vi "Transport To Actor Type.vi"(10 "Spawn":refnum<class "Spawn.lvclass">) -> (2 "Actor Type":T1)   [LabVIEW 2025, in "jettl.lvlib" / "Actor.lvlib"]
uses:
  Actor.lvlib
  Actor Type.ctl
  Transport/Queue/Queue.lvlib
  Transport/Event/Event.lvlib
  Transport/Notifier/Notifier.lvlib
  Spawn/Spawn/Spawn.lvclass
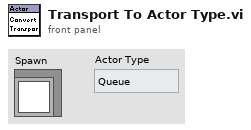
[diagram p1: front panel]
types:
  T1 = typedef "jettl.lvlib/Actor.lvlib/Actor Type.ctl" = enum16{"Queue", "Event", "Notifier"}
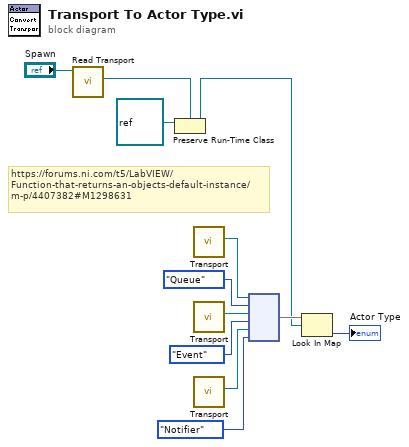
[diagram p0: block diagram]
diagram:
  # "https://forums.ni.com/t5/LabVIEW/Function-that-returns-an-objects-default-instance/m-p/4407382#M1298631"
  n1 = call-dynamic "Read Transport.vi"("Spawn in"="Spawn") -> ("Transport"=w2:refnum<class "Transport.lvclass">)  [unwired: 10 in]
  n2 = Preserve Run-Time Class(object in=refnum<class> refnum ("LabVIEW Object"), 2:w2) -> (object out=w4:refnum<class "Transport.lvclass">)  [unwired: 1 in, 1 out]
  n3 = call "Transport.vi"() -> ("Transport"=w12:refnum<class "Transport.lvclass">)  [unwired: 11 in]
  n4 = call "Transport.vi"() -> ("Transport"=w10:refnum<class "Transport.lvclass">)  [unwired: 11 in]
  n5 = call "Transport.vi"() -> ("Transport"=w9:refnum<class "Transport.lvclass">)  [unwired: 11 in]
  n6 = node(w12, Actor_Type."Queue" ("Actor Type"), w10, Actor_Type."Event" ("Actor Type"), w9, Actor_Type."Notifier" ("Actor Type")) -> (w6:map{refnum<class "Transport.lvclass">, T1})
  n7 = Look In Map(map=w6, key=w4) -> (value=→"Actor Type":T1)  [unwired: 1 in, 1 out]
